vi "军蚁-引导算角度3.vi"(7 "error in":errorcluster) -> (27 "error out":errorcluster)   [LabVIEW 2015]
uses:
  <vilib>/vision/Pattern Matching.llb/IMAQ Curve Parameters.ctl
  <vilib>/vision/Pattern Matching.llb/IMAQ Match Range Setting.ctl
  <vilib>/vision/Measure.llb/Straight Edge Options.ctl
  <vilib>/vision/Measure.llb/Straight Edge Process.ctl
  <vilib>/vision/Measure.llb/Edge Options.ctl
  <vilib>/vision/Measure.llb/Edge Polarity.ctl
  <vilib>/vision/NI_Vision_Development_Module.lvlib
panel:
  out "Image Out":T1(plugin-control)
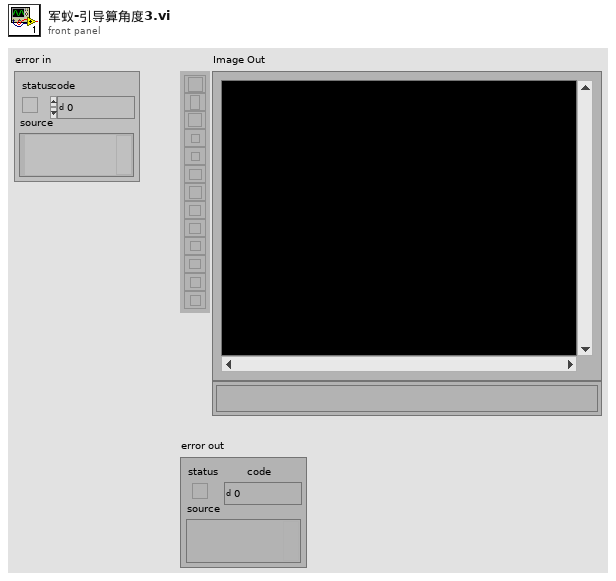
[diagram p1: front panel]
types:
  T1 = typedef "IMAQ Image.ctl" = refnum<image>
  T2 = typedef "Edge Options.ctl" = cluster{"Edge Polarity":T3, "Kernel Size":u32, "Width":u32, "Minimum Edge Strength":sgl, "Interpolation Type":enum32{"Zero Order", "Bilinear", "Quadratic", "Cubic", "Bilinear Fixed"}, "Data Processing Method":enum32{"Average", "Median"}}
  T3 = typedef "Edge Polarity.ctl" = u32
  T4 = cluster{"Search Direction":u32, "Edge Options":T2, "Show Search Area":bool, "Show Search Lines":bool, "Show Edges Found":bool, "Show Result":bool, "Search Area Color":u32, "Search Lines Color":u32, "Edge Locations Color":u32, "Result Color":u32, "Overlay Group Name":string}
  T5 = typedef "Straight Edge Options.ctl" = cluster{"Number of Lines":i32, "Type":T6, "Min. Score":dbl, "Max. Score":dbl, "Orientation":dbl, "Angle Range":dbl, "Angle Tolerance":dbl, "Step Size":u32, "Min. SNR (db)":dbl, "Min. Points (%)":dbl, "Hough Iterations":i32}
  T6 = typedef "Straight Edge Process.ctl" = enum32{"First Edge Rake", "Best Edge Rake", "Hough Edge Rake", "First Edge Projection", "Best Edge Projection"}
  T7 = cluster{"Global Rectangle":i32[], "Contours":cluster{"ID":enum32{"External", "Internal"}, "Type":u32, "Coordinates":i32[]}[]}
  T8 = cluster{"Origin":cluster{"X":sgl, "Y":sgl}, "Angle (deg)":sgl, "Axis Reference":u32}
  T9 = enum16{"Reset", "Update Coordinate System", "Get Coordinate System"}
  T10 = enum16{"Horizontal Motion", "Vertical Motion", "Horizontal and Vertical Motion", "Horizontal, Vertical and Angular Motion"}
  T11 = typedef "IMAQ Curve Parameters.ctl" = cluster{"Extraction Mode":u32, "Edge Threshold":i32, "Edge Filter Size":u32, "Min Length":i32, "Row Search Step Size":i32, "Col Search Step Size":i32, "Max Endpoint Gap":i32, "Closed":bool, "Subpixel":bool}
  T12 = typedef "IMAQ Match Range Setting.ctl" = cluster{"Match Constraints":u32, "Min":dbl, "Max":dbl}
  T13 = cluster{"Curve Parameters":T11, "Match Mode":cluster{"Rotation":bool, "Scale":bool, "Occlusion":bool, "Reserved":bool, "Reserved":bool, "Reserved":bool}, "Range Settings":T12[], "Number of Matches":i32, "Minimum Match Score":sgl, "SubPixel Accuracy":bool, "Adv. Geometric Match Options 2":cluster{"Setup Data Item":u16, "Item Value":dbl}[]}
  T14 = typedef "Image Type" = u32
  T15 = typedef "IMAQ GM Match Report.ctl" = cluster{"Position":cluster{"x":sgl, "y":sgl}, "Angle":sgl, "Scale":sgl, "Score":sgl, "Bounding Box":cluster{"x":sgl, "y":sgl}[], "Contrast Reversed":bool, "Occlusion %":sgl, "Template Target Curve Score":sgl, "Target Template Curve Score":sgl, "Correlation Score":sgl}
  T16 = typedef "IMAQ Coordinate System" = cluster{"Reference System":cluster{"Origin":cluster{"X":sgl, "Y":sgl}, "Angle (deg)":sgl, "Axis Reference":u32}, "Measurement System":cluster{"Origin":cluster{"X":sgl, "Y":sgl}, "Angle (deg)":sgl, "Axis Reference":u32}}
  T17 = typedef "ROI Descriptor" = cluster{"Global Rectangle":i32[], "Contours":cluster{"ID":enum32{"External", "Internal"}, "Type":u32, "Coordinates":i32[]}[]}
  T18 = cluster{"Point1 (Pixels)":cluster{"X":sgl, "Y":sgl}, "Point2 (Pixels)":cluster{"X":sgl, "Y":sgl}, "Point1 (Real-World)":cluster{"X":sgl, "Y":sgl}, "Point2 (Real-World)":cluster{"X":sgl, "Y":sgl}, "Angle (Pixel)":dbl, "Angle (Real-World)":dbl, "Score":dbl, "Straightness":dbl, "Average SNR (db)":dbl, "Calibration Valid":bool}[]
  T19 = cluster{"Point1 (Pixels)":cluster{"X":sgl, "Y":sgl}, "Point2 (Pixels)":cluster{"X":sgl, "Y":sgl}, "Point1 (Real-World)":cluster{"X":sgl, "Y":sgl}, "Point2 (Real-World)":cluster{"X":sgl, "Y":sgl}, "Angle (Pixel)":dbl, "Angle (Real-World)":dbl, "Score":dbl, "Straightness":dbl, "Average SNR (db)":dbl, "Calibration Valid":bool}
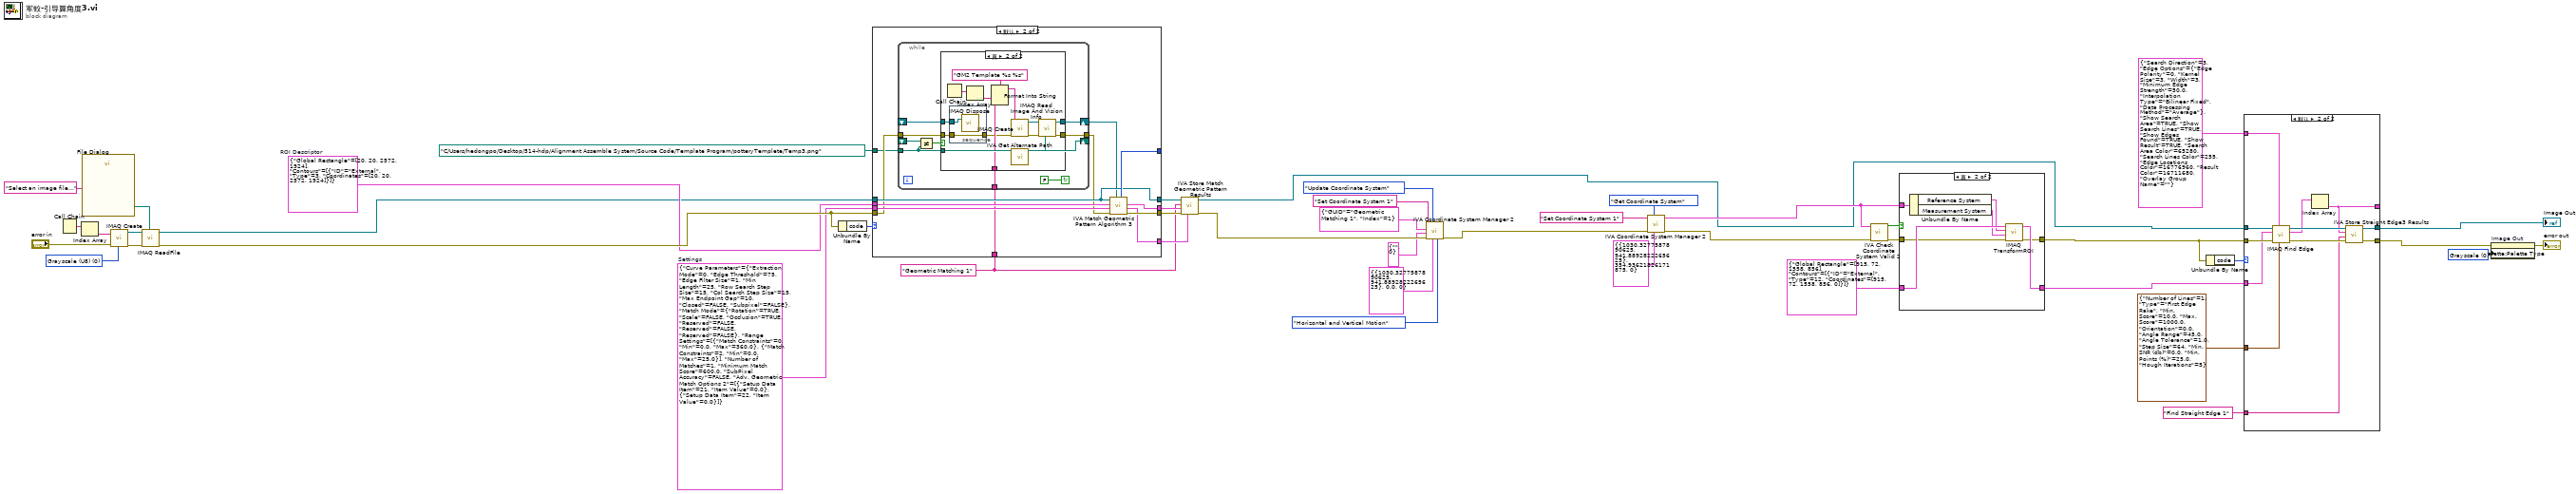
[diagram p0: block diagram]
diagram:
  w1 = u32 0 items=["Grayscale", "Binary", "Gradient", "Rainbow", "Temperature", "User Defined", "Binary 16 Bit", "Gradient 16 Bit", "Rainbow 16 Bit", "Temperature 16 Bit", "User Defined 16 Bit"] ("Palette Type")
  w28 = T13 {"Curve Parameters"={"Extraction Mode"=0, "Edge Threshold"=75, "Edge Filter Size"=1, "Min Length"=25, "Row Search Step Size"=15, "Col Search Step Size"=15, "Max Endpoint Gap"=10, "Closed"=FALSE, "Subpixel"=FALSE}, "Match Mode"={"Rotation"=TRUE, "Scale"=FALSE, "Occlusion"=TRUE, "Reserved"=FALSE, "Reserved"=FALSE, "Reserved"=FALSE}, "Range Settings"=[{"Match Constraints"=0, "Min"=0.0, "Max"=360.0}, {"Match Constraints"=2, "Min"=0.0, "Max"=25.0}], "Number of Matches"=1, "Minimum Match Score"=600.0, "SubPixel Accuracy"=FALSE, "Adv. Geometric Match Options 2"=[{"Setup Data Item"=21, "Item Value"=0.0}, {"Setup Data Item"=22, "Item Value"=0.0}]}  # Settings
  w27 = "Geometric Matching 1" ("Step Name")
  w36 = T7 {"Global Rectangle"=[20, 20, 2572, 1924], "Contours"=[{"ID"=enum."External", "Type"=3, "Coordinates"=[20, 20, 2572, 1924]}]}  # ROI Descriptor
  w38 = T14 0 items=["Grayscale (U8)", "Grayscale (I16)", "Grayscale (SGL)", "Complex (CSG)", "RGB (U32)", "HSL (U32)", "RGB (U64)", "Grayscale (U16)"] ("Image Type")
  n1 = Call Chain() -> (call chain=w42:string[])
  n2 = Index Array(array=w42) -> (element=w41:string)  [unwired: 1 in]
  n3 = call "File Dialog"("prompt"="Select an image file...") -> ("selected path"=w39:path)  [unwired: 6 in, 8 out]
  n4 = call "IMAQ Create"("Image Name"=w41, "Image Type"=w38, "error in (no error)"="error in") -> ("New Image"=w45:T1, "error out"=w44:errorcluster)  [unwired: 1 in, 1 out]
  n5 = call "IMAQ ReadFile"("File Path"=w39, "error in (no error)"=w44, "Image"=w45) -> ("error out"=w46:errorcluster, "Image Out"=w35:T1)  [unwired: 2 in, 5 out]
  n6 = Unbundle By Name(w46) -> ("code"=w30:i32)
  n7 = case "条件结构" shown="默认" w30 {
    tunnel: path "C:/Users/hedongpo/Desktop/514-hdp/Alignment Assemble System/Source Code/Template Program/potteryTemplete/Temp3.png" ("Template File Path") -> [_ w49]
    tunnel: w46 -> [_ w50]
    tunnel: w28 -> [_ w59]
    tunnel: w36 -> [_ w58]
    tunnel: w35 -> [w47 w53]
    tunnel: [_ w57] -> w34
    tunnel: [_ w56] -> w32
    tunnel: [_ w55] -> w31
    tunnel: [_ w54] -> _
    tunnel: [w47 w53] -> w29
    tunnel: w27 -> [_ w48]
    frame -1074396199, -1074396198 {
      # "Discard Coordinate System Error"
    }
    frame Default {
      n8 = while {
        shift-right: [w68] -> w51
        shift-left: _ -> [w67]
        tunnel: [w65] -> w52
        tunnel: w50 -> [w64]
        tunnel: w49 -> [w60]
        tunnel: w48 -> [w63]
        shift-right: [w60] -> _
        shift-left: _ -> [w62]
        stop <- FALSE continue-if-true
        n9 = Not Equal?(x=w62, y=w60) -> (x != y?=w61:bool)
        n10 = case "条件结构" shown="真" w61 {
          tunnel: [w70 w82] -> w68
          tunnel: w67 -> [w70 w74]
          tunnel: [w69 w79] -> w65
          tunnel: w64 -> [w69 w75]
          tunnel: w63 -> [_ w76]
          tunnel: w60 -> [_ w72]
          frame False {
          }
          frame True {
            n11 = Call Chain() -> (call chain=w78:string[])
            n12 = stacked-sequence "层叠式顺序结构" {
              tunnel: w75 -> [w86]
              tunnel: w74 -> [w85]
              tunnel: [w86] -> w73
              frame #0 {
                n13 = call "IMAQ Dispose"("Image"=w85) -> ()  [unwired: 2 in, 4 out]
              }
            }
            n14 = Index Array(array=w78) -> (element=w77:string)  [unwired: 1 in]
            n15 = Format Into String(format string="GM2 Template %s %s" ("Image Name"), w77, w76) -> (resulting string=w84:string)  [unwired: 2 in, 1 out]
            n16 = call "IMAQ Create"("Image Name"=w84, "error in (no error)"=w73) -> ("New Image"=w81:T1, "error out"=w80:errorcluster)  [unwired: 2 in, 1 out]
            n17 = call <vilib>:"IVA Get Alternate Path.vi"("Path In"=w72) -> ("Path Out"=w71:path)  [unwired: 10 out]
            n18 = call "IMAQ Read Image And Vision Info"("File Path"=w71, "error in (no error)"=w80, "Image"=w81) -> ("error out"=w79:errorcluster, "Image Out"=w82:T1)  [unwired: 1 in, 6 out]
          }
        }
      }
      n19 = call <vilib>:"IVA Match Geometric Pattern Algorithm 3.vi"("Template"=w51, "error in (no error)"=w52, "Settings"=w59, "ROI Descriptor"=w58, "Image"=w53) -> ("error out"=w57:errorcluster, "Calibrated Matches"=w55:T15[], "Matches"=w56:T15[], "Number of Matches"=w54:i32)  [unwired: 3 out]
    }
  }
  n20 = call <vilib>:"IVA Store Match Geometric Pattern Results.vi"("Calibrated Matches"=w31, "error in (no error)"=w34, "Matches"=w32, "Step Name"=w27, "Image in"=w29) -> ("error out"=w33:errorcluster, "Image dup"=w10:T1)  [unwired: 5 out]
  n21 = call <vilib>:"IVA Coordinate System Manager 2.vi"("Mode"=T10."Horizontal and Vertical Motion", "Reference System"=T8 {"Origin"={"X"=1030.3278, "Y"=941.8893}, "Angle (deg)"=0.0, "Axis Reference"=0}, "Function"=T9."Update Coordinate System", "error in (no error)"=w33, "Angle ID"=cluster{"GUID":string, "Index":i32} {"GUID"="", "Index"=0}, "Origin ID"=cluster{"GUID":string, "Index":i32} {"GUID"="Geometric Matching 1", "Index"=1}, "Coordinate System Name"="Set Coordinate System 1") -> ("error out"=w20:errorcluster)  [unwired: 4 out]
  n22 = call <vilib>:"IVA Coordinate System Manager 2.vi"("Reference System"=T8 {"Origin"={"X"=1030.3278, "Y"=941.8893}, "Angle (deg)"=354.93622, "Axis Reference"=0}, "Function"=T9."Get Coordinate System", "error in (no error)"=w20, "Coordinate System Name"="Set Coordinate System 1") -> ("error out"=w17:errorcluster, "Coordinate System Out"=w13:T16)  [unwired: 3 in, 3 out]
  n23 = call <vilib>:"IVA Check Coordinate System Valid 2.vi"("error in (no error)"=w17, "Coordinate System"=w13) -> ("error out"=w11:errorcluster, "Valid?"=w12:bool)  [unwired: 8 out]
  n24 = case "条件结构" shown="真" w12 {
    tunnel: T7 {"Global Rectangle"=[915, 72, 1558, 856], "Contours"=[{"ID"=enum."External", "Type"=12, "Coordinates"=[915, 72, 1558, 856, 0]}]} ("ROI Descriptor") -> [w88 w95]
    tunnel: [w88 w92] -> w9
    tunnel: [w87 w91] -> w14
    tunnel: w13 -> [_ w90]
    tunnel: w11 -> [w87 w89]
    frame False {
    }
    frame True {
      n25 = Unbundle By Name(w90) -> ("Reference System"=w94:T8, "Measurement System"=w93:T8)
      n26 = call "IMAQ TransformROI"("error in (no error)"=w89, "New Reference"=w93, "Base Reference"=w94, "ROI Descriptor"=w95) -> ("error out"=w91:errorcluster, "ROI Descriptor out"=w92:T17)  [unwired: 6 out]
    }
  }
  n27 = Unbundle By Name(w14) -> ("code"=w6:i32)
  n28 = case "条件结构" shown="默认" w6 {
    tunnel: w10 -> [w96 w108]
    tunnel: w14 -> [_ w107]
    tunnel: w9 -> [_ w101]
    tunnel: [w96 w105] -> w2
    tunnel: [_ w103] -> w8
    tunnel: "Find Straight Edge 1" ("Step Name") -> [_ w102]
    tunnel: T5 {"Number of Lines"=1, "Type"=enum."First Edge Rake", "Min. Score"=10.0, "Max. Score"=1000.0, "Orientation"=0.0, "Angle Range"=45.0, "Angle Tolerance"=1.0, "Step Size"=64, "Min. SNR (db)"=0.0, "Min. Points (%)"=25.0, "Hough Iterations"=5} ("Fit Options") -> [_ w100]
    tunnel: T4 {"Search Direction"=3, "Edge Options"={"Edge Polarity"=0, "Kernel Size"=3, "Width"=3, "Minimum Edge Strength"=50.0, "Interpolation Type"=enum."Bilinear Fixed", "Data Processing Method"=enum."Average"}, "Show Search Area"=TRUE, "Show Search Lines"=TRUE, "Show Edges Found"=TRUE, "Show Result"=TRUE, "Search Area Color"=65280, "Search Lines Color"=255, "Edge Locations Color"=16776960, "Result Color"=16711680, "Overlay Group Name"=""} ("Options") -> [_ w99]
    tunnel: [_ w97] -> _
    frame -1074396199, -1074396198 {
      # "Discard Coordinate System Error"
    }
    frame Default {
      n29 = call "IMAQ Find Edge"("Line Fit Options"=w100, "Options"=w99, "error in (no error)"=w107, "ROI Descriptor"=w101, "Image"=w108) -> ("error out"=w104:errorcluster, "Straight Edges"=w98:T18, "Image Out"=w106:T1)  [unwired: 1 in, 3 out]
      n30 = Index Array(array=w98) -> (element=w97:T19)  [unwired: 1 in]
      n31 = call <vilib>:"IVA Store Straight Edge3 Results.vi"("error in (no error)"=w104, "Step Name"=w102, "Straight Edge"=w97, "Image in"=w106) -> ("error out"=w103:errorcluster, "Image dup"=w105:T1)  [unwired: 1 in, 5 out]
    }
  }
  "Image Out" <- w2
  n32 = property on="Image Out" class="ImageControl"(error in=w8, "Palette:Palette Type"=w1) -> (error out=→"error out":errorcluster)  [unwired: 1 in, 1 out]
